vi "clone.vi"(0 "reference in":refnum<class "VINode.lvclass">, 5 "error in (no error)":errorcluster) -> (14 "reference out":refnum<class "VINode.lvclass">, 15 "clonedClassNode":refnum<class "AbstractNode.lvclass">, 19 "error out":errorcluster)   [LabVIEW 2020, in "VINode.lvclass"]
doc: "public Object clone()"
uses:
  <resource>/Framework/Providers/Open_GDS/UML/VINode_class/VINode.lvclass
  C:/Program Files (x86)/National Instruments/LabVIEW 2020/resource/Framework/Providers/Open_GDS/UML/RectangularNode_class/RectangularNode.lvclass
  C:/Program Files (x86)/National Instruments/LabVIEW 2020/resource/Framework/Providers/Open_GDS/UML/AbstractNode_class/AbstractNode.lvclass
  <resource>/Framework/Providers/Open_GDS/UML/AbstractNode_class/AbstractNode.lvclass
  <resource>/Framework/Providers/Open_GDS/UML/MultiLineString_class/MultiLineString.lvclass
  <resource>/Framework/Providers/Open_GDS/UML/RectangularNode_class/RectangularNode.lvclass
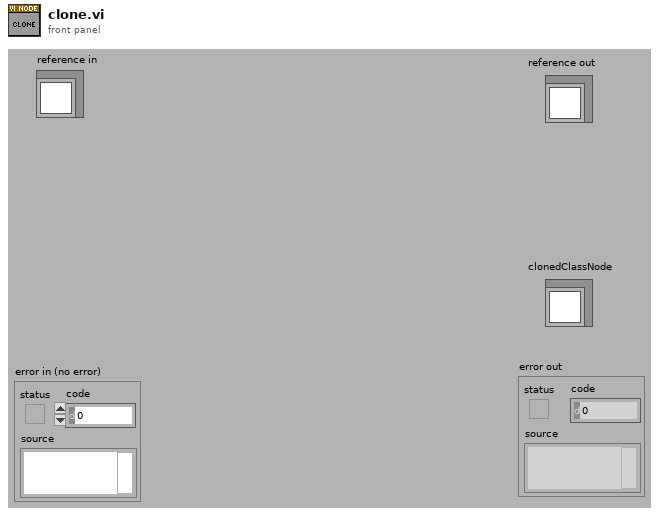
[diagram p1: front panel]
types:
  T1 = typedef "RectangularNode.lvclass/ObjectAttributes.ctl" = cluster{"bounds":T2}
  T2 = typedef "Rectangle Rectangle2D.ctl" = cluster{"x":dbl, "y":dbl, "width":dbl, "height":dbl}
  T3 = typedef "VINode.lvclass/ObjectAttributes.ctl" = cluster{"midHeight":dbl, "botHeight":dbl, "Name":refnum<class "MultiLineString.lvclass">, "DEFAULT_COMPARTMENT_HEIGHT":i32, "DEFAULT_WIDTH":i32, "DEFAULT_HEIGHT":i32, "VIPath":path, "Description":refnum<class "MultiLineString.lvclass">, "ShowDescription":bool}
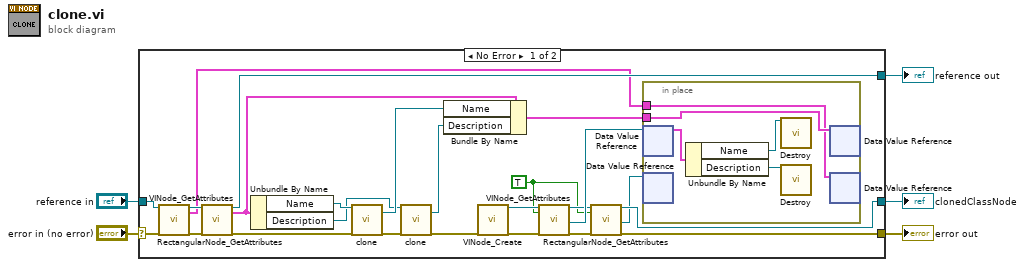
[diagram p0: block diagram]
diagram:
  n1 = case shown="No Error" "error in (no error)" {
    selector: "error in (no error)" -> [w29 w35]
    tunnel: "reference in" -> [w13 w36]
    tunnel: [w11 w35] -> w4
    tunnel: [w23 w36] -> w3
    tunnel: [w9 _] -> w1
    frame No Error {
      w6 = TRUE ("OnlyGetDvrReference(False)")
      n2 = call <resource>:"RectangularNode_GetAttributes.vi"("reference in"=w13, "error in (no error)"=w29) -> ("reference out"=w12:refnum<class "VINode.lvclass">, "Data"=w7:T1, "error out"=w14:errorcluster)  [unwired: 14 in, 1 out]
      n3 = call <resource>:"VINode_GetAttributes.vi"("reference in"=w12, "error in (no error)"=w14) -> ("reference out"=w23:refnum<class "VINode.lvclass">, "Data"=w22:T3, "error out"=w26:errorcluster)  [unwired: 1 in, 14 out]
      n4 = Unbundle By Name(w22) -> ("Name"=w28:refnum<class "MultiLineString.lvclass">, "Description"=w16:refnum<class "MultiLineString.lvclass">)
      n5 = call-dynamic "clone.vi"("reference"=w28, "error in (no error)"=w26) -> ("clonedMultiLineString"=w27:refnum<class "MultiLineString.lvclass">, "error out"=w18:errorcluster)  [unwired: 15 in, 1 out]
      n6 = call-dynamic "clone.vi"("reference"=w16, "error in (no error)"=w18) -> ("clonedMultiLineString"=w15:refnum<class "MultiLineString.lvclass">, "error out"=w17:errorcluster)  [unwired: 15 in, 1 out]
      n7 = Bundle By Name(cluster=w22, "Name"=w27, "Description"=w15) -> (w19:T3)
      n8 = call <resource>:"VINode_Create.vi"("error in (no error)"=w17) -> ("reference out"=w25:refnum<class "VINode.lvclass">, "error out"=w24:errorcluster)  [unwired: 17 in]
      n9 = call <resource>:"VINode_GetAttributes.vi"("reference in"=w25, "OnlyGetDvrReference(False)"=w6, "error in (no error)"=w24) -> ("reference out"=w10:refnum<class "VINode.lvclass">, "DataRef"=w20:refnum<data-value>, "error out"=w21:errorcluster)  [unwired: 13 in, 1 out]
      n10 = call <resource>:"RectangularNode_GetAttributes.vi"("reference in"=w10, "OnlyGetDvrReference(False)"=w6, "error in (no error)"=w21) -> ("reference out"=w9:refnum<class "VINode.lvclass">, "DataRef"=w8:refnum<data-value>, "error out"=w11:errorcluster)  [unwired: 13 in, 1 out]
      n11 = in-place {
        in-place-border: w19 -> [w34]
        in-place-border: w7 -> [w30]
        n12 = in-place-dvr #1(w20) -> (w32:T3)  [unwired: 1 out]
        n13 = in-place-dvr #2(w8) -> ()  [unwired: 2 out]
        n14 = Unbundle By Name(w32) -> ("Name"=w33:refnum<class "MultiLineString.lvclass">, "Description"=w31:refnum<class "MultiLineString.lvclass">)
        n15 = call-dynamic "Destroy.vi"("reference"=w33) -> ()  [unwired: 17 in, 2 out]
        n16 = call-dynamic "Destroy.vi"("reference"=w31) -> ()  [unwired: 17 in, 2 out]
        n17 = in-place-dvr #1(w34) -> ()  [unwired: 2 out]
        n18 = in-place-dvr #2(w30) -> ()  [unwired: 2 out]
      }
    }
    frame Error {
    }
  }
  "reference out" <- w3
  "error out" <- w4
  "clonedClassNode" <- w1
